vi "Miroir.vi"(11 "Pixel":u8[](array[numeric])) -> (3 "Pixel Miroir":u8[](array[numeric]))   [LabVIEW 2014]
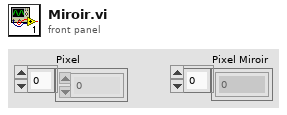
[diagram p1: front panel]
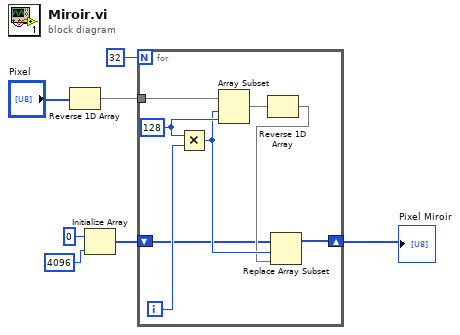
[diagram p0: block diagram]
diagram:
  n1 = Reverse 1D Array(array="Pixel") -> (reversed array=w5:u8[])
  n2 = Initialize Array(u8 0, 4096) -> (w2:u8[])
  n3 = for {
    N: 32 -> [_]
    tunnel: w5 -> [w15]
    shift-right: [w8] -> w1
    shift-left: w2 -> [w9]
    i -> [w13]
    w14 = 128
    n4 = Multiply(x=w14, y=w13) -> (x*y=w11:i32)
    n5 = Array Subset(array=w15, index=w11, length=w14) -> (w12:u8[])
    n6 = Reverse 1D Array(array=w12) -> (reversed array=w10:u8[])
    n7 = Replace Array Subset(array=w9, new element=w10, index=w11) -> (w8:u8[])
  }
  "Pixel Miroir" <- w1
